vi "Test App Shutdown Process.vi"(8 "error in (no error)":errorcluster, 11 "Rig Test in":refnum<class "Application Test.lvclass">) -> (0 "error out":errorcluster, 3 "Rig Test out":refnum<class "Application Test.lvclass">)   [LabVIEW 2020, in "Application Test.lvclass"]
uses:
  Application Test.lvclass
  C:/Program Files (x86)/National Instruments/LabVIEW 2020/vi.lib/Astemes/LUnit/Test Case.lvclass
  Framework/Process/Process.lvclass
  Framework/Process/Public/Lifecycle/Lifecycle State.ctl
  Framework/Process/Process.lvclass/Process.ctl
  Framework/Application/Application.lvclass/Application.ctl
  <vilib>/Astemes/LUnit/Test Case.lvclass/Test Case.ctl
  <vilib>/Astemes/LUnit/LUnit Assertion Result.lvclass/LUnit Assertion Result.ctl
  <vilib>/Astemes/LUnit/LUnit Test Case Result.lvclass/LUnit Test Case Result.ctl
  <vilib>/Astemes/LUnit/LUnit Method Result.lvclass/LUnit Method Result.ctl
  Framework/Application/Private/Add Process to Map.vi
  Framework/Application/Private/Start Idle Processes if Running.vi
  Framework/Application/Private/Throw Error If Process Already in App.vi
  Framework/Process/Protected/Messaging/Enqueue Message.vi
  Framework/Process/Public/Lifecycle/Get Lifecycle State.vi
  Framework/Process/Protected/SubVIs/Set Context.vi
  Framework/Application/Private/Remove Process from Map.vi
  <vilib>/Astemes/LUnit/Set Assertion Type.vi
  <vilib>/Astemes/LUnit/Palette/Pass.vi
  <vilib>/Astemes/LUnit/Palette/Fail.vi
  Framework/Process/Private/SubVIs/Wait for finish.vi
  Framework/Process/Private/SubVIs/Set Lifecycle State.vi
  Framework/Application/Public/Get Process.vi
  Framework/Process/Private/SubVIs/Handle Debug Data.vi
  <vilib>/Utility/error.llb/Clear Errors.vi
  Framework/Process/Public/Lifecycle/Leave Process Loop.vi
  <vilib>/Astemes/LUnit/LUnit Write Assertion Type.vi
  <vilib>/Astemes/LUnit/Add test result.vi
  <vilib>/Astemes/LUnit/LUnit Write Passed.vi
  <vilib>/Astemes/LUnit/LUnit Write Message.vi
  <vilib>/Astemes/LUnit/LUnit Write Description.vi
  Framework/Application/Private/Retrieve Process from App.vi
  Framework/Application/Private/Parse Process Name.vi
  Framework/Application/Private/Get Process from Map.vi
  Framework/Logging/Log Debug.vi
  <vilib>/AdvancedString/1D String Array to Delimited String.vi
  <vilib>/Utility/High Resolution Relative Seconds.vi
  <vilib>/Astemes/LUnit/LUnit Record Assertion Result.vi
  Framework/Process/Protected/Messaging/Request Message.vi
  <vilib>/AdvancedString/Delimited String to 1D String Array.vi
  <vilib>/Astemes/LUnit/LUnit Aggregate Assertion Results.vi
  Framework/Process/Private/SubVIs/Enqueue Request Message.vi
  <vilib>/Astemes/LUnit/Assertion Result/LUnit Read Status.vi
  <vilib>/Astemes/LUnit/LUnit Read Message.vi
  <vilib>/Astemes/LUnit/LUnit Read Description.vi
  <vilib>/Astemes/LUnit/Method Result/LUnit Merge Status.vi
  <vilib>/Astemes/LUnit/LUnit Concatenate result strings.vi
  Framework/Application/Application.lvclass
  C:/Git/astemes-triarc-framework/source/Framework/Process/Process.lvclass
  <vilib>/Utility/error.llb/Error Cluster From Error Code.vi
  Framework/Process/Public/Read Name.vi
  Framework/Process/Private/SubVIs/Wait for Response Message.vi
  <vilib>/Astemes/LUnit/LUnit Assertion Result.lvclass
  Application Test.lvclass/Application Test.ctl
  <vilib>/Astemes/LUnit/Test Case.lvclass
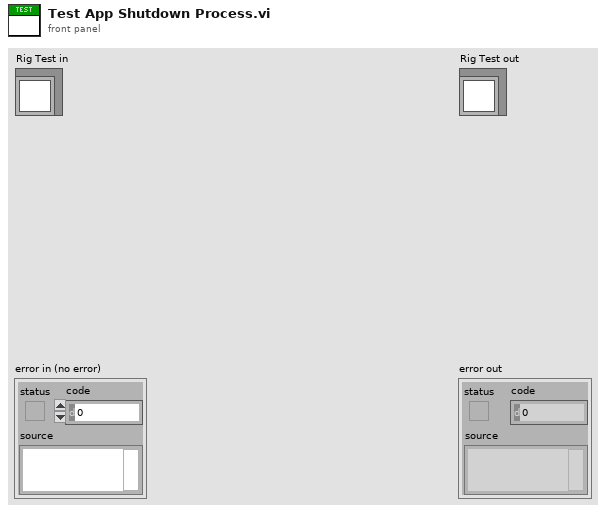
[diagram p1: front panel]
types:
  T1 = typedef "Process.lvclass/Lifecycle State.ctl" = enum16{"Uninitialized", "Initialized", "Started", "Running", "Stopped", "Finished"}
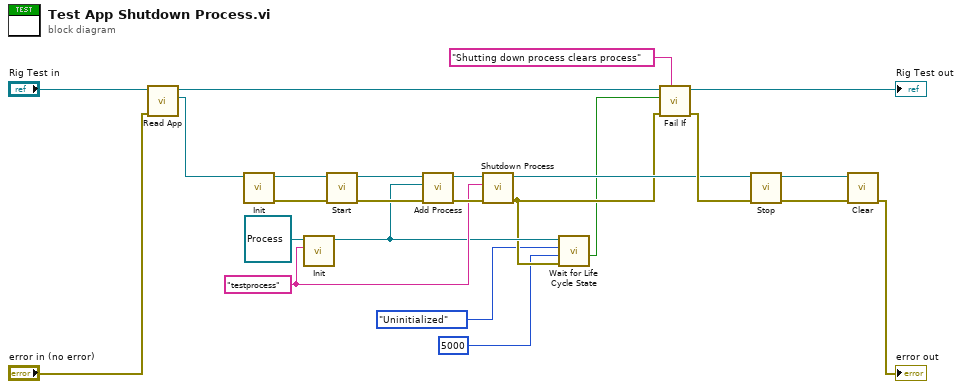
[diagram p0: block diagram]
diagram:
  w6 = "testprocess" ("Name")
  n1 = call "Read App.vi"("error in (no error)"="error in (no error)", "Application Test In"="Rig Test in") -> ("App out"=w23:refnum<class "Application.lvclass">, "Application Test Out"=w12:refnum<class "Application Test.lvclass">)  [unwired: 7 in, 1 out]
  n2 = call-dynamic "Init.vi"("Process In"=w23) -> ("error out"=w13:errorcluster, "Process Out"=w14:refnum<class "Application.lvclass">)  [unwired: 9 in]
  n3 = call-dynamic "Init.vi"("Name"=w6, "Process In"=refnum<class "Process.lvclass"> refnum ("Process.lvclass")) -> ("Process Out"=w5:refnum<class "Process.lvclass">)  [unwired: 8 in, 1 out]
  n4 = call "Start.vi"("error in (no error)"=w13, "Process In"=w14) -> ("error out"=w15:errorcluster, "Process Out"=w16:refnum<class "Application.lvclass">)  [unwired: 7 in, 1 out]
  n5 = call "Add Process.vi"("error in (no error)"=w15, "Process"=w5, "Application In"=w16) -> ("error out"=w20:errorcluster, "Application Out"=w8:refnum<class "Application.lvclass">)  [unwired: 7 in]
  n6 = call "Shutdown Process.vi"("error in (no error)"=w20, "Process Name"=w6, "Application In"=w8) -> ("error out"=w4:errorcluster, "Application Out"=w7:refnum<class "Application.lvclass">)  [unwired: 7 in]
  n7 = call "Wait for Life Cycle State.vi"("error in (no error)"=w4, "timeout in ms (-1)"=5000, "Lifecycle State"=Lifecycle_State."Uninitialized", "Process In"=w5) -> ("timed out?"=w1:bool)  [unwired: 5 in, 2 out]
  n8 = call <vilib>:"Fail If.vi"("Description"="Shutting down process clears process", "error in (no error)"=w4, "Fail?"=w1, "LUnit Test Case In"=w12) -> ("error out"=w18:errorcluster, "LUnit Test Case Out"=→"Rig Test out":refnum<class "Application Test.lvclass">)  [unwired: 6 in]
  n9 = call "Stop.vi"("error in (no error)"=w18, "Process In"=w7) -> ("error out"=w11:errorcluster, "Process Out"=w10:refnum<class "Application.lvclass">)  [unwired: 7 in, 1 out]
  n10 = call-dynamic "Clear.vi"("error in (no error)"=w11, "Application In"=w10) -> ("error out"=→"error out":errorcluster)  [unwired: 9 in]
